vi "SetS0Bit.vi"(8 "error in (no error)":errorcluster, 9 "Address":u8, 10 "bitnumber":u32, 11 "board_sel":u32) -> (0 "error out":errorcluster)   [LabVIEW 2015, in "ESLSCDLL.lvlib"]
uses:
  ESLSCDLL.lvlib
  ESLSCDLL.dll
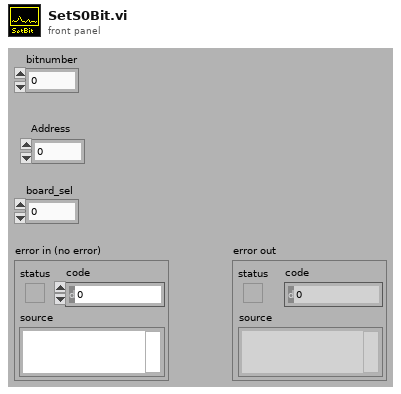
[diagram p1: front panel]
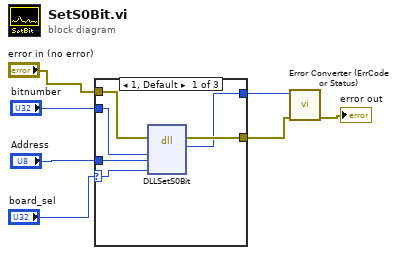
[diagram p0: block diagram]
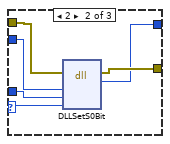
[diagram p2: hidden frame]
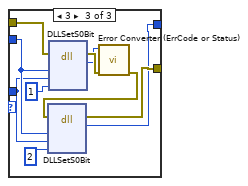
[diagram p3: hidden frame]
diagram:
  n1 = case shown="1, Default" "board_sel" {
    selector: "board_sel" -> [w13 w17 _]
    tunnel: "Address" -> [w12 w18 w28]
    tunnel: "bitnumber" -> [w11 w19 w29]
    tunnel: "error in (no error)" -> [w10 w16 w25]
    tunnel: [w9 w15 w21] -> w2
    tunnel: [w8 w14 w20] -> w1
    frame 1, Default {
      n2 = dll-call lib="C:/Users/flori/Nextcloud/Dokumente/Stresing/Windows/lv64/board.vis/ESLSCDLL.dll" fn="DLLSetS0Bit" ("lwlscdll.dll:DLLRsTOREG")(error in=w10, "bitnumber"=w11, "Address"=w12, "drv"=w13) -> (error out=w9:errorcluster, "es_status_codes"=w8:i32)  [unwired: 5 in, 1 out]
    }
    frame 2 {
      n3 = dll-call lib="C:/Users/flori/Nextcloud/Dokumente/Stresing/Windows/lv64/board.vis/ESLSCDLL.dll" fn="DLLSetS0Bit" ("lwlscdll.dll:DLLRsTOREG")(error in=w16, "bitnumber"=w19, "Address"=w18, "drv"=w17) -> (error out=w15:errorcluster, "es_status_codes"=w14:i32)  [unwired: 5 in, 1 out]
    }
    frame 3 {
      n4 = dll-call lib="C:/Users/flori/Nextcloud/Dokumente/Stresing/Windows/lv64/board.vis/ESLSCDLL.dll" fn="DLLSetS0Bit" ("lwlscdll.dll:DLLRsTOREG")(error in=w25, "bitnumber"=w29, "Address"=w28, "drv"=u32 1) -> (error out=w24:errorcluster, "es_status_codes"=w23:i32)  [unwired: 5 in, 1 out]
      n5 = call "Error Converter (ErrCode or Status).vi"("error in (no error)"=w24, "error code"=w23) -> ("error out"=w22:errorcluster)  [unwired: 9 in]
      n6 = dll-call lib="C:/Users/flori/Nextcloud/Dokumente/Stresing/Windows/lv64/board.vis/ESLSCDLL.dll" fn="DLLSetS0Bit" ("lwlscdll.dll:DLLRsTOREG")(error in=w22, "bitnumber"=w29, "Address"=w28, "drv"=u32 2) -> (error out=w21:errorcluster, "es_status_codes"=w20:i32)  [unwired: 5 in, 1 out]
    }
  }
  n7 = call "Error Converter (ErrCode or Status).vi"("error in (no error)"=w2, "error code"=w1) -> ("error out"=→"error out":errorcluster)  [unwired: 9 in]
